vi "Secure WebSocket Client Test with dotNET.vi"() -> ()   [LabVIEW 2013]
uses:
  dotNET SSL Socket/dotNET WebSocket/Client/SSL Client Options.ctl
  dotNET SSL Socket/dotNET SSL Socket/PFX Certificate.ctl
  dotNET SSL Socket/dotNET WebSocket/Client/dotNET WebSocket Client.lvclass
  <vilib>/MediaMongrels Ltd/WebSockets/WebSockets/WebSocket/WebSocket.lvclass/WebSocket.ctl
  <vilib>/MediaMongrels Ltd/WebSockets/WebSockets/WebSocket/Read Return Headers.vi
  <vilib>/MediaMongrels Ltd/WebSockets/WebSockets/WebSocket Client/WebSocket Client.lvclass
  dotNET SSL Socket/dotNET SSL Client/dotNET SSL Client Socket.lvclass
  dotNET SSL Socket/dotNET TCP Socket/dotNET TCP Socket.lvclass
  dotNET SSL Socket/dotNET SSL Socket/dotNET SSL Socket.lvclass
panel:
  out "Array":string[](array[string])
  out "error out":errorcluster
  out "Return Headers 2":variant
  out "Data 2":string
  out "Data":string
  out "Return Headers":variant
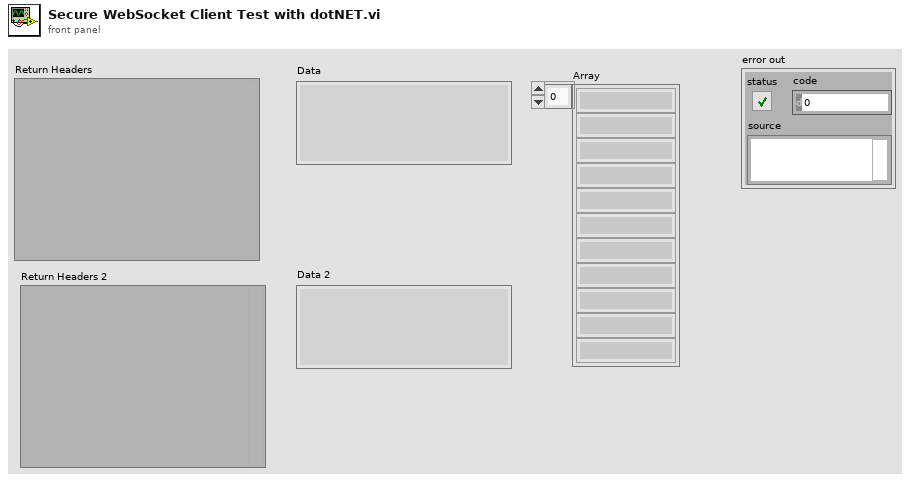
[diagram p1: front panel]
types:
  T1 = typedef "dotNET WebSocket.lvlib/dotNET WebSocket Client.lvclass/SSL Client Options.ctl" = cluster{"Check Revocation":bool, "SSL Protocols":i32[], "Client Certs":T2[]}
  T2 = typedef "dotNET SSL Socket.lvlib/dotNET SSL Socket.lvclass/PFX Certificate.ctl" = cluster{"PFX Certificate":path, "PFX Password":string}
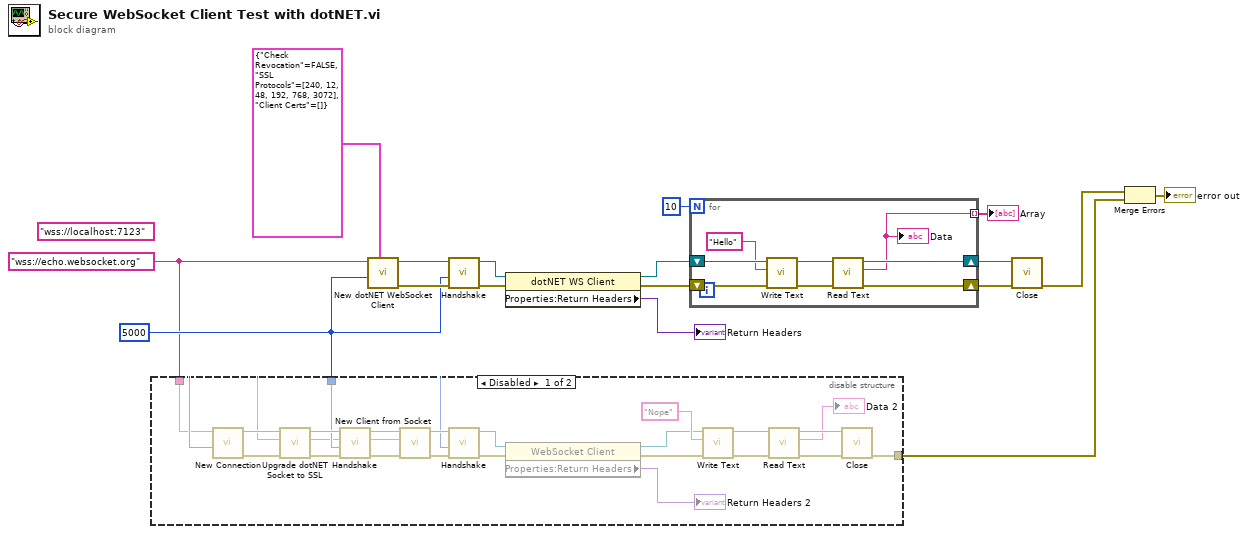
[diagram p0: block diagram]
diagram:
  (unwired) "wss://localhost:7123" ("WebSocket URL")
  w5 = 5000 ("Timeout (5000ms)")
  w3 = "wss://echo.websocket.org" ("WebSocket URL")
  n1 = disable-structure shown="Disabled" {
    disable-tunnel: [w39 _] -> w9
    disable-tunnel: w5 -> [w19 _]
    disable-tunnel: w3 -> [w18 _]
    frame Disabled {
      n2 = call "New Connection.vi"("Timeout (5000ms)"=w19, "Hostname / URL"=w18) -> ("error out"=w20:errorcluster, "dotNET TCP Socket out"=w24:refnum<class "dotNET TCP Socket.lvclass">)  [unwired: 8 in]
      n3 = call "Upgrade dotNET Socket to SSL.vi"("error in (no error)"=w20, "Hostname / URL"=w18, "dotNET TCP Socket in"=w24) -> ("error out"=w21:errorcluster, "dotNET SSL Client Socket out"=w25:refnum<class "dotNET SSL Client Socket.lvclass">)  [unwired: 7 in]
      n4 = call-dynamic "Handshake.vi"("error in (no error)"=w21, "Timeout (5000ms)"=w19, "dotNET SSL Client Socket in"=w25) -> ("error out"=w22:errorcluster, "dotNET SSL Client Socket out"=w23:refnum<class "dotNET SSL Client Socket.lvclass">)  [unwired: 7 in]
      n5 = call <vilib>:"New Client from Socket.vi"("error in (no error)"=w22, "WebSocket URL"=w18, "Socket in"=w23) -> ("error out"=w26:errorcluster, "WebSocket Client out"=w27:refnum<class "WebSocket Client.lvclass">)  [unwired: 7 in]
      n6 = call-dynamic "Handshake.vi"("error in (no error)"=w26, "timeout ms (5000)"=w19, "WebSocket Client in"=w27) -> ("error out"=w28:errorcluster, "WebSocket Client out"=w29:refnum<class "WebSocket Client.lvclass">)  [unwired: 7 in]
      n7 = property class="WebSocket Client"(reference=w29, error in=w28) -> (reference out=w32:refnum<class "WebSocket Client.lvclass">, error out=w31:errorcluster, "Properties:Return Headers"=→"Return Headers 2":variant)
      n8 = call-dynamic "Write Text.vi"("error in (no error)"=w31, "String Data"="Nope", "WebSocket in"=w32) -> ("error out"=w34:errorcluster, "WebSocket out"=w35:refnum<class "WebSocket Client.lvclass">)  [unwired: 7 in]
      n9 = call-dynamic "Read Text.vi"("error in (no error)"=w34, "WebSocket in"=w35) -> ("error out"=w37:errorcluster, "Data"=→"Data 2":string, "WebSocket out"=w38:refnum<class "WebSocket Client.lvclass">)  [unwired: 7 in]
      n10 = call-dynamic "Close.vi"("error in (no error)"=w37, "WebSocket in"=w38) -> ("error out"=w39:errorcluster)  [unwired: 9 in]
    }
    frame Enabled {
    }
  }
  n11 = call "New dotNET WebSocket Client.vi"("Client SSL Options (wss://)"=T1 {"Check Revocation"=FALSE, "SSL Protocols"=[240, 12, 48, 192, 768, 3072], "Client Certs"=[]} ("SSL Options (for wss://)"), "Timeout (5000ms)"=w5, "WebSocket URL"=w3) -> ("error out"=w7:errorcluster, "dotNET WS Client out"=w6:refnum<class "dotNET WebSocket Client.lvclass">)  [unwired: 7 in]
  n12 = call-dynamic "Handshake.vi"("error in (no error)"=w7, "timeout ms (5000)"=w5, "WebSocket Client in"=w6) -> ("error out"=w17:errorcluster, "WebSocket Client out"=w16:refnum<class "dotNET WebSocket Client.lvclass">)  [unwired: 7 in]
  n13 = property class="dotNET WS Client"(reference=w16, error in=w17) -> (reference out=w13:refnum<class "dotNET WebSocket Client.lvclass">, error out=w14:errorcluster, "Properties:Return Headers"=→"Return Headers":variant)
  n14 = for {
    N: 10 -> [_]
    shift-right: [w41] -> w11
    shift-left: w13 -> [w46]
    shift-right: [w42] -> w12
    shift-left: w14 -> [w47]
    tunnel: [w40] -> w2 mode=indexing
    n15 = call-dynamic "Write Text.vi"("error in (no error)"=w47, "String Data"="Hello", "WebSocket in"=w46) -> ("error out"=w44:errorcluster, "WebSocket out"=w43:refnum<class "dotNET WebSocket Client.lvclass">)  [unwired: 7 in]
    n16 = call-dynamic "Read Text.vi"("error in (no error)"=w44, "WebSocket in"=w43) -> ("error out"=w42:errorcluster, "Data"=w40:string, "WebSocket out"=w41:refnum<class "dotNET WebSocket Client.lvclass">)  [unwired: 7 in]
    "Data" <- w40
  }
  "Array" <- w2
  n17 = call-dynamic "Close.vi"("error in (no error)"=w12, "WebSocket in"=w11) -> ("error out"=w10:errorcluster)  [unwired: 9 in]
  n18 = Merge Errors(w10, w9) -> (→"error out":errorcluster)
